vi "UHR-Fleezers Control (host) - 11.1.vi"() -> ()   [LabVIEW 2012] (continued)
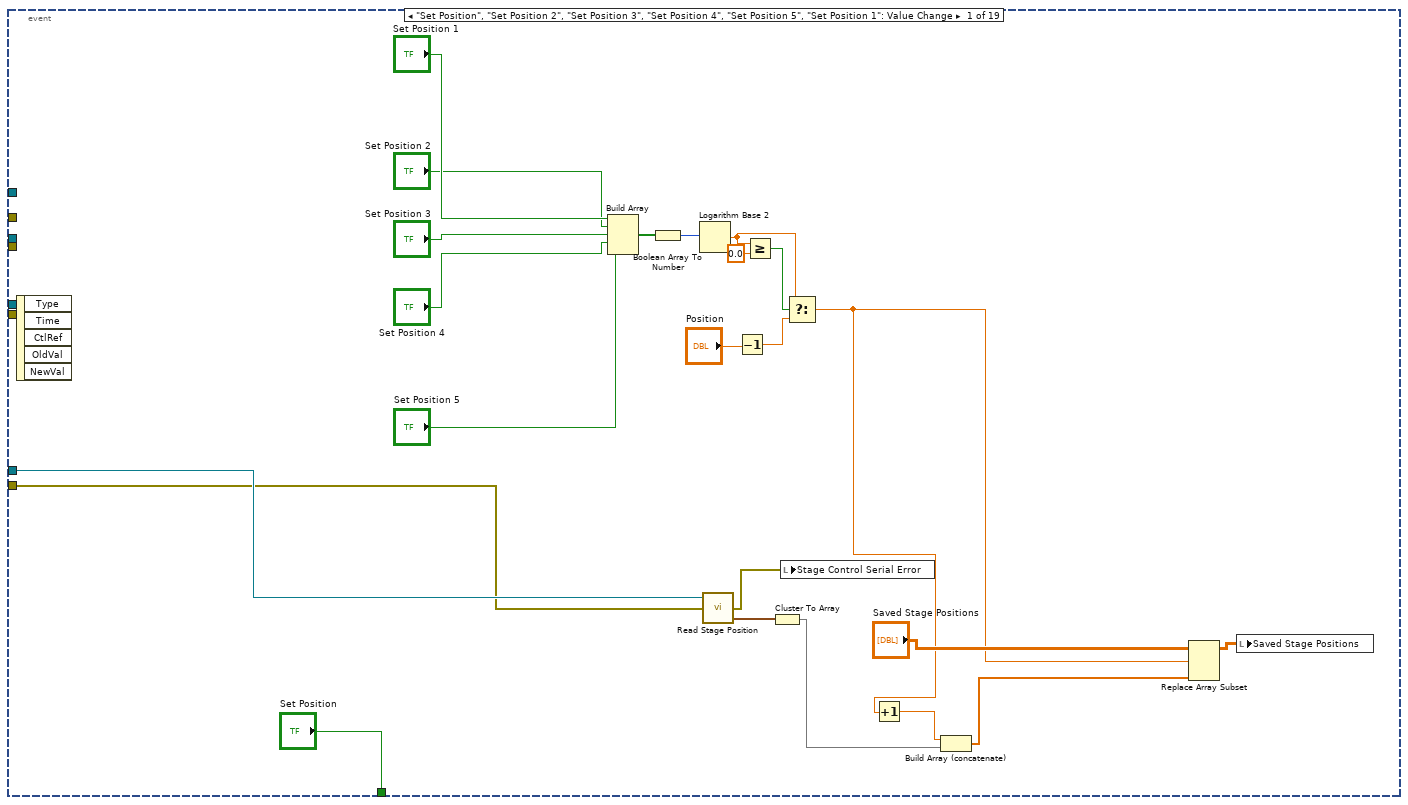
[diagram p2: hidden frame]
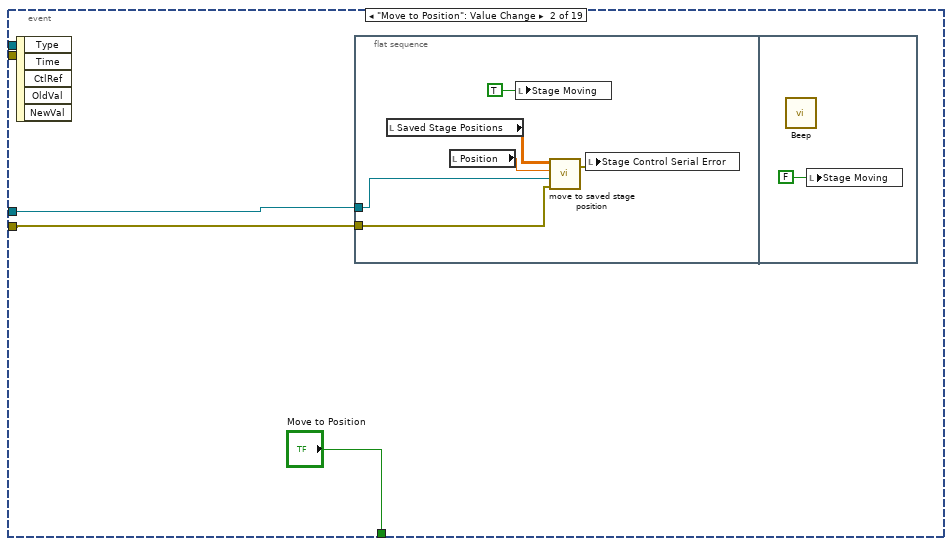
[diagram p3: hidden frame]
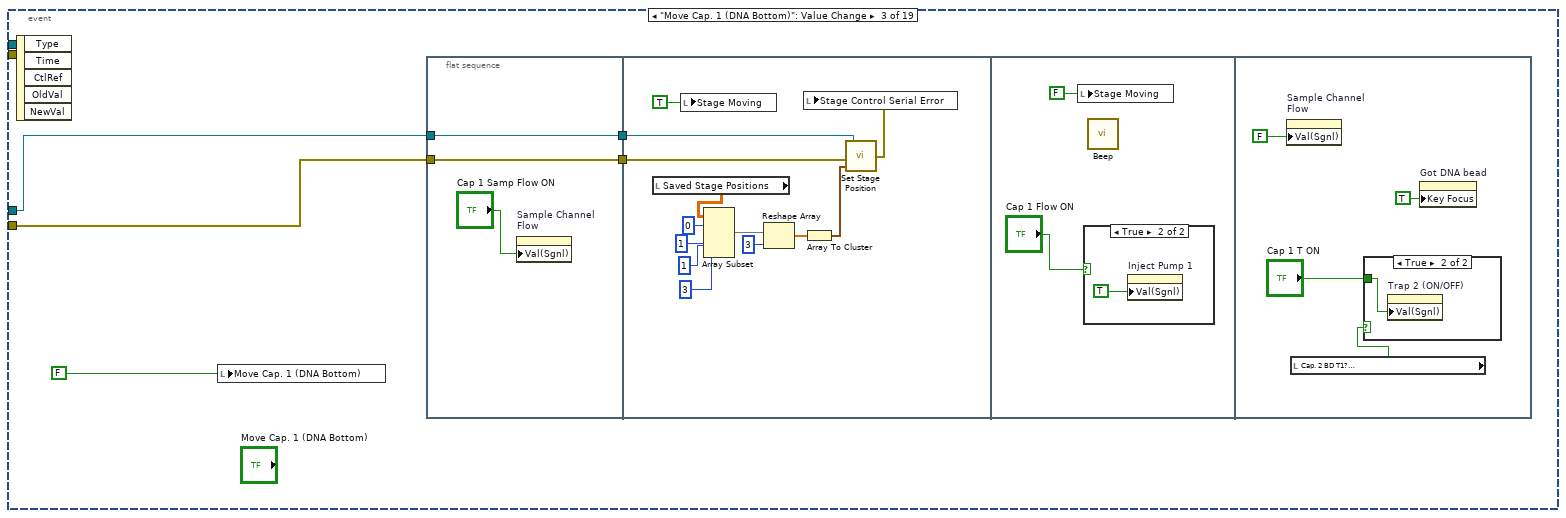
[diagram p4: hidden frame]
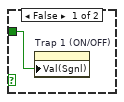
[diagram p6: hidden frame]
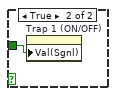
[diagram p8: hidden frame]
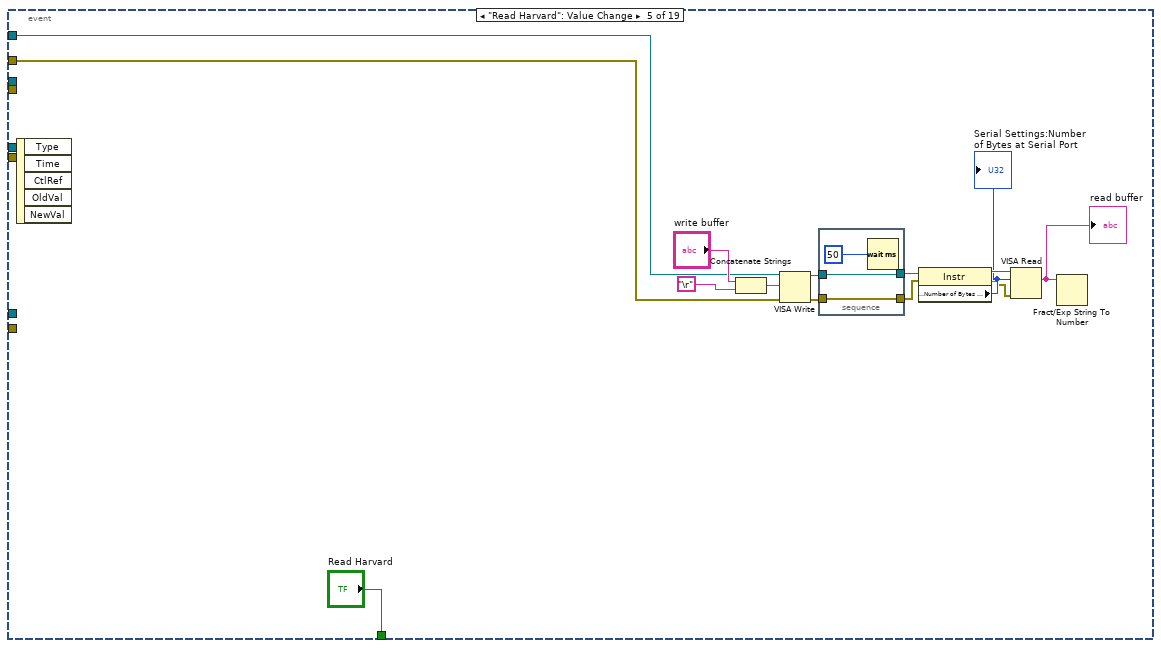
[diagram p9: hidden frame]
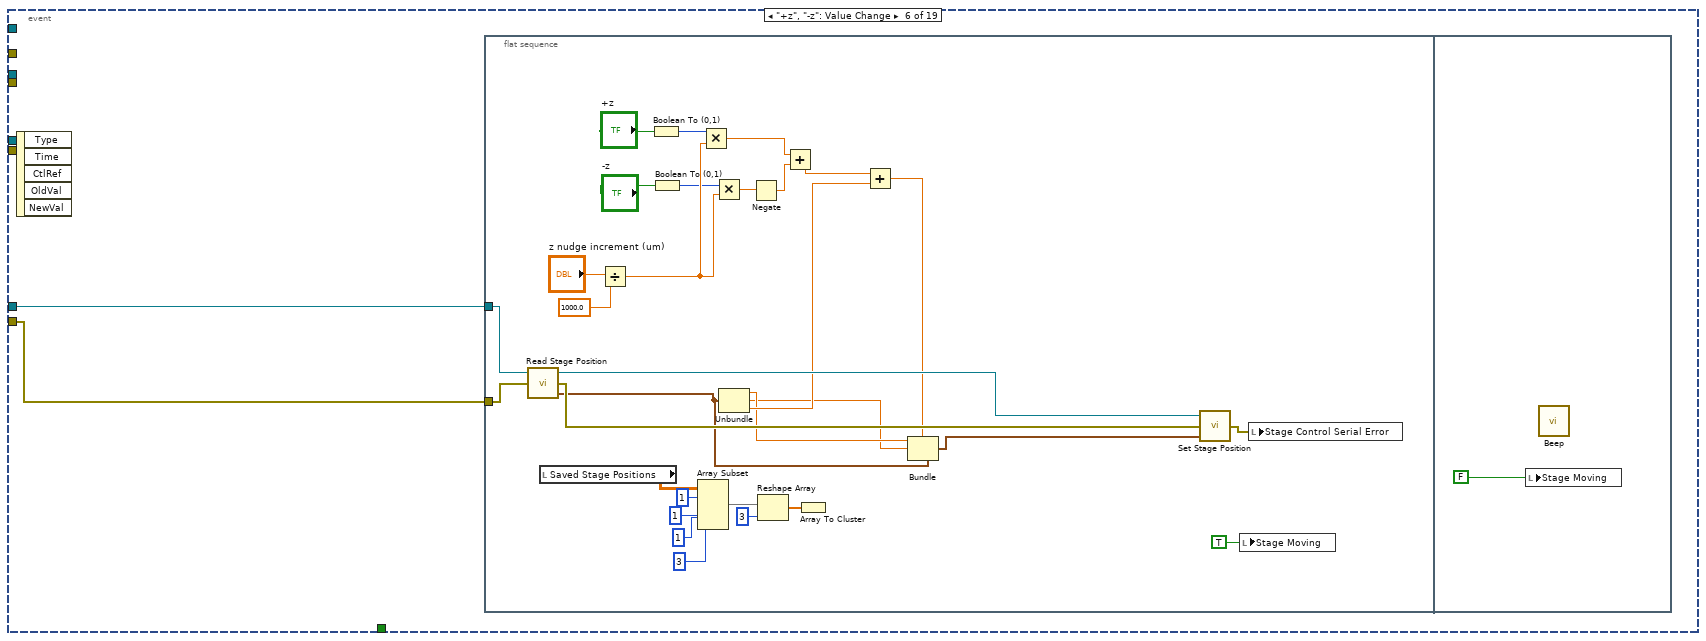
[diagram p10: hidden frame]
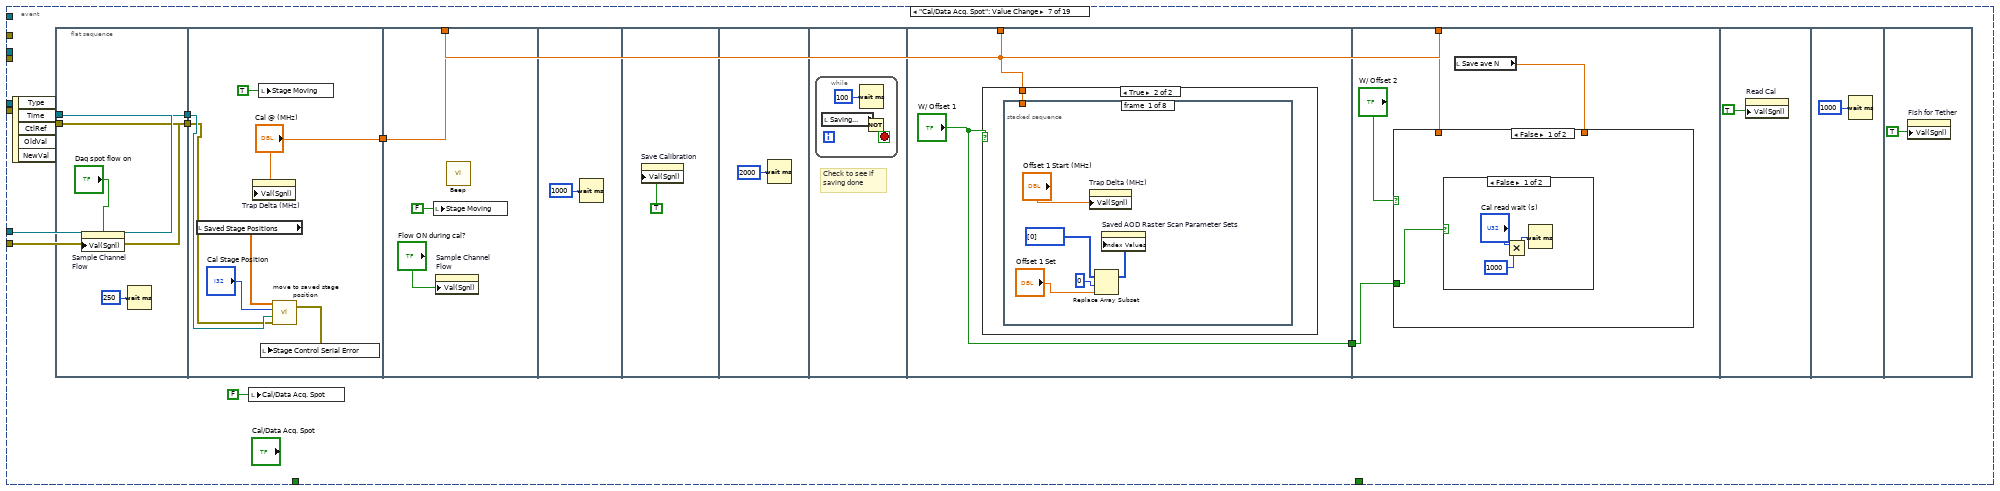
[diagram p11: hidden frame]
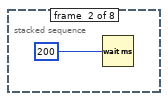
[diagram p13: hidden frame]
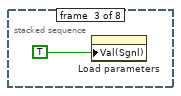
[diagram p14: hidden frame]
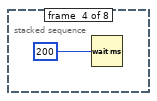
[diagram p15: hidden frame]
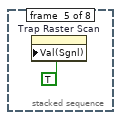
[diagram p16: hidden frame]
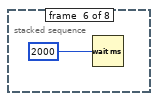
[diagram p17: hidden frame]
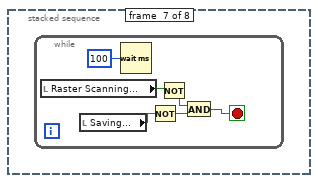
[diagram p18: hidden frame]
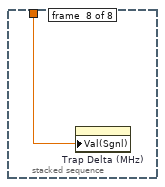
[diagram p19: hidden frame]
                                frame True {
                                n2888 = local read "Confocal Y 1 (V)"() -> (w4656:dbl)
                                n2889 = local read "Confocal X 1 (V)"() -> (w4655:dbl)
                                n2890 = property on="AO2" class="Slide (strict)"("Val(Sgnl)"=w4655) -> ()  [unwired: 2 in, 2 out]
                                n2891 = property on="AO1" class="Slide (strict)"("Val(Sgnl)"=w4656) -> ()  [unwired: 2 in, 2 out]
                                }
                                }
                                }
                                }
                                }
                                }
                                }
                                }
                                }
                                }
                                n2892 = local read "Time (s)"() -> (w4593:dbl)
                                n2893 = Subtract(x=w4594, y=w4593) -> (x-y=w4605:dbl)
                                n2894 = Number To Decimal String(number=w4605, width (-)=i16 0) -> (decimal integer string=w4603:string)
                                n2895 = Concatenate Strings(w4603, " s fluorescence event") -> (w4600:string)
                                n2896 = local read "Messages"() -> (w4601:string)
                                n2897 = local write "Duration (s)"(w4605) -> ()
                                n2898 = call "Update messages.vi"("Message to add"=w4600, "Old message string"=w4601) -> ("New message string"=w4599:string)
                                n2899 = local write "Messages"(w4599) -> ()
                                n2900 = call <vilib>:"Beep.vi"() -> ()  [unwired: 12 in]
                                n2901 = local write "Reset Force"(FALSE ("Force Reset")) -> ()
                                n2902 = local write "Fl. High"(TRUE ("Fl. High")) -> ()
                                n2903 = local write "Waiting"(TRUE ("Waiting")) -> ()
                                }
                                }
                                n2904 = node-c288() -> ()  [unwired: 1 in, 1 out]
                                }
                                n2905 = node-c288(w4572) -> ()  [unwired: 1 out]
                                }
                              }
                            }
                          }
                          n2906 = local read "Trap Delta (MHz)"() -> (w4484:dbl)
                          n2907 = local read "Trap Pos FB SP"() -> (w4482:fxp<+/-,16,1>)
                        }
                      }
                    }
                    frame True {
                      n2908 = flat-sequence {
                        tunnel: w4669 -> [w4679]
                        tunnel: [w4679] -> w4673
                        tunnel: w4672 -> [w4678]
                        tunnel: [w4678] -> w4671
                        tunnel: [w4677] -> w4670
                        tunnel: w4668 -> [w4676]
                        tunnel: [w4675] -> w4667
                        tunnel: w4664 -> [w4674]
                        tunnel: [w4674] -> w4663
                        tunnel: w4673 -> [w4749]
                        tunnel: w4671 -> [w4748]
                        tunnel: w4670 -> [w4747]
                        tunnel: w4667 -> [w4746]
                        tunnel: w4663 -> [w4745]
                        tunnel: [w4746] -> w4666
                        frame #0 {
                          n2909 = call <vilib>:"Beep.vi"() -> ()  [unwired: 3 in, 9 out]
                          n2910 = local write "Waiting"(FALSE ("Waiting")) -> ()
                          n2911 = Increment(x=w4676) -> (x+1=w4675:u8)
                          n2912 = case shown="\"Yank\"" w4678 {
                            tunnel: w4675 -> [_ _ w4685]
                            frame "Image" {
                              n2913 = property on="Confocal Image" class="Bool (strict)"("Val(Sgnl)"=TRUE ("Value (Signaling)")) -> ()  [unwired: 2 in, 2 out]
                            }
                            frame "Alarm", Default {
                            }
                            frame "Yank" {
                              n2914 = flat-sequence {
                                tunnel: w4685 -> [w4688]
                                tunnel: [w4687] -> w4684
                                tunnel: ["N Array El"] -> w4683
                                tunnel: w4684 -> [w4702]
                                tunnel: w4683 -> [w4698]
                                frame #0 {
                                n2915 = Multiply(x="Yank Delay (s)", y=1000.0) -> (x*y=w4691:dbl)
                                n2916 = Quotient & Remainder(x=w4688, y="N Array El") -> (x-y*floor(x/y)=w4687:u8)  [unwired: 1 out]
                                n2917 = Wait (ms)(milliseconds to wait=w4691) -> ()  [unwired: 1 out]
                                }
                                frame #1 {
                                n2918 = Random Number (0-1)() -> (number: 0 to 1=w4699:dbl)
                                n2919 = Multiply(x=w4698, y=w4699) -> (x*y=w4697:dbl)
                                n2920 = Round Toward -Infinity(1:w4697) -> (0:w4696:dbl)
                                n2921 = Select(t=w4696, s="Random Choice", f=w4702) -> (s? t:f=w4700:dbl)
                                n2922 = Select(t="Yank to Trap Delta (MHz)", s="Yank to which?", f="Yank to SP") -> (s? t:f=w4693:dbl[])
                                n2923 = Index Array(array=w4693, index=w4700) -> (element=w4703:dbl)
                                n2924 = case shown="False" "Yank to which?" {
                                tunnel: w4703 -> [w4704 w4730]
                                frame False {
                                n2925 = flat-sequence {
                                tunnel: w4704 -> [w4705]
                                frame #0 {
                                n2926 = property on="Trap Pos FB SP" class="DigNum (strict)"("Val(Sgnl)"=w4705) -> ()  [unwired: 2 in, 2 out]
                                }
                                frame #1 {
                                n2927 = Wait (ms)(milliseconds to wait=u32 700) -> ()  [unwired: 1 out]
                                }
                                frame #2 {
                                n2928 = local read "Action (%)"() -> (w4710:dbl)
                                n2929 = Absolute Value(x=w4710) -> (abs(x)=w4709:dbl)
                                n2930 = Greater?(x=w4709, y=70.0) -> (0:w4707:bool)
                                n2931 = property on="Remove Action Offset" class="Bool (strict)"("Val(Sgnl)"=w4707) -> ()  [unwired: 2 in, 2 out]
                                }
                                frame #3 {
                                n2932 = for {
                                N: 4 -> [_]
                                n2933 = flat-sequence {
                                frame #0 {
                                n2934 = Wait (ms)(milliseconds to wait=u32 500) -> ()  [unwired: 1 out]
                                }
                                frame #1 {
                                n2935 = local read "Action (%)"() -> (w4716:dbl)
                                n2936 = Absolute Value(x=w4716) -> (abs(x)=w4715:dbl)
                                n2937 = Greater?(x=w4715, y=70.0) -> (0:w4713:bool)
                                n2938 = property on="Remove Action Offset" class="Bool (strict)"("Val(Sgnl)"=w4713) -> ()  [unwired: 2 in, 2 out]
                                }
                                }
                                }
                                }
                                frame #4 {
                                n2939 = local read "Shift confocal"() -> (w4720:bool)
                                n2940 = local read "Mean"() -> (w4723:dbl)
                                n2941 = Greater?(x=w4723, y=11.0) -> (0:w4719:bool)
                                n2942 = Not(x=w4719) -> (.not. x?=w4718:bool)
                                n2943 = And(x=w4718, y=w4720) -> (x .and. y?=w4717:bool)
                                n2944 = And(x=w4719, y=w4720) -> (x .and. y?=w4721:bool)
                                n2945 = case shown="True" w4721 {
                                frame False {
                                }
                                frame True {
                                n2946 = local read "Confocal X 2 (V)"() -> (w4726:dbl)
                                n2947 = local read "Confocal Y 2 (V)"() -> (w4727:dbl)
                                n2948 = property on="AO2" class="Slide (strict)"("Val(Sgnl)"=w4726) -> ()  [unwired: 2 in, 2 out]
                                n2949 = property on="AO1" class="Slide (strict)"("Val(Sgnl)"=w4727) -> ()  [unwired: 2 in, 2 out]
                                }
                                }
                                n2950 = case shown="True" w4717 {
                                frame False {
                                }
                                frame True {
                                n2951 = local read "Confocal X 1 (V)"() -> (w4724:dbl)
                                n2952 = local read "Confocal Y 1 (V)"() -> (w4725:dbl)
                                n2953 = property on="AO1" class="Slide (strict)"("Val(Sgnl)"=w4725) -> ()  [unwired: 2 in, 2 out]
                                n2954 = property on="AO2" class="Slide (strict)"("Val(Sgnl)"=w4724) -> ()  [unwired: 2 in, 2 out]
                                }
                                }
                                }
                                frame #5 {
                                n2955 = Wait (ms)(milliseconds to wait=u32 1500) -> ()  [unwired: 1 out]
                                }
                                frame #6 {
                                n2956 = property on="Rem fb disp offset" class="Bool (strict)"("Val(Sgnl)"=TRUE ("Value (Signaling)")) -> ()  [unwired: 2 in, 2 out]
                                }
                                }
                                }
                                frame True {
                                n2957 = flat-sequence {
                                tunnel: w4730 -> [w4731]
                                frame #0 {
                                n2958 = property on="Trap Delta (MHz)" class="DigNum (strict)"("Val(Sgnl)"=w4731) -> ()  [unwired: 2 in, 2 out]
                                }
                                frame #1 {
                                n2959 = Wait (ms)(milliseconds to wait=u32 500) -> ()  [unwired: 1 out]
                                }
                                frame #2 {
                                n2960 = local read "Shift confocal"() -> (w4735:bool)
                                n2961 = local read "Mean"() -> (w4733:dbl)
                                n2962 = Greater?(x=w4733, y=11.0) -> (0:w4736:bool)
                                n2963 = Not(x=w4736) -> (.not. x?=w4737:bool)
                                n2964 = And(x=w4737, y=w4735) -> (x .and. y?=w4739:bool)
                                n2965 = And(x=w4736, y=w4735) -> (x .and. y?=w4738:bool)
                                n2966 = case shown="True" w4738 {
                                frame False {
                                }
                                frame True {
                                n2967 = local read "Confocal Y 2 (V)"() -> (w4743:dbl)
                                n2968 = local read "Confocal X 2 (V)"() -> (w4742:dbl)
                                n2969 = property on="AO1" class="Slide (strict)"("Val(Sgnl)"=w4743) -> ()  [unwired: 2 in, 2 out]
                                n2970 = property on="AO2" class="Slide (strict)"("Val(Sgnl)"=w4742) -> ()  [unwired: 2 in, 2 out]
                                }
                                }
                                n2971 = case shown="True" w4739 {
                                frame False {
                                }
                                frame True {
                                n2972 = local read "Confocal X 1 (V)"() -> (w4740:dbl)
                                n2973 = local read "Confocal Y 1 (V)"() -> (w4741:dbl)
                                n2974 = property on="AO2" class="Slide (strict)"("Val(Sgnl)"=w4740) -> ()  [unwired: 2 in, 2 out]
                                n2975 = property on="AO1" class="Slide (strict)"("Val(Sgnl)"=w4741) -> ()  [unwired: 2 in, 2 out]
                                }
                                }
                                }
                                }
                                }
                                }
                                }
                              }
                            }
                          }
                          n2976 = local read "Time (s)"() -> (w4677:dbl)
                          "Fl. High" <- TRUE ("Yanking")
                        }
                        frame #1 {
                          n2977 = local read "Auto F Reset"() -> (w4744:bool)
                          n2978 = case shown="True" w4744 {
                            tunnel: w4749 -> [_ w4753]
                            tunnel: w4748 -> [_ w4752]
                            tunnel: w4747 -> [_ w4751]
                            tunnel: w4745 -> [_ w4750]
                            frame False {
                            }
                            frame True {
                              n2979 = node-c288() -> (w4755:T21)  [unwired: 4 out]
                              n2980 = timed-loop {
                                timing: w4755 -> [_]
                                timing-out: [_] -> w4754
                                tunnel: w4753 -> [w4773]
                                tunnel: w4752 -> [w4772]
                                tunnel: w4751 -> [w4771]
                                tunnel: w4750 -> [w4770]
                                stop <- w4756 stop-if-true
                                n2981 = node-c288() -> ()  [unwired: 2 out]
                                n2982 = local read "Fl. Delta Thresh. (kHz)"() -> (w4764:dbl)
                                n2983 = local read "Fl. Triggered..."() -> (w4769:bool)
                                n2984 = local read "Delta Fl. 1"() -> (w4760:dbl)
                                n2985 = local read "Delta Fl. 2"() -> (w4758:dbl)
                                n2986 = local read "Stop All"() -> (w4767:bool)
                                n2987 = local read "APD to Watch"() -> (w4759:bool)
                                n2988 = Select(t=w4760, s=w4759, f=w4758) -> (s? t:f=w4757:dbl)
                                n2989 = Not(x=w4769) -> (.not. x?=w4768:bool)
                                n2990 = Multiply(x=w4764, y=1000.0) -> (x*y=w4763:dbl)
                                n2991 = Negate(x=w4763) -> (-x=w4762:dbl)
                                n2992 = Less?(x=w4757, y=w4762) -> (x < y?=w4766:bool)
                                n2993 = Compound Arithmetic op=OR(w4766, w4767, w4768, "Reset Force") -> (w4756:bool)
                                n2994 = case shown="True" w4756 {
                                tunnel: w4773 -> [_ w4788]
                                tunnel: w4772 -> [_ w4787]
                                tunnel: w4771 -> [_ w4777]
                                tunnel: w4770 -> [_ w4779]
                                frame False {
                                }
                                frame True {
                                n2995 = local read "Time (s)"() -> (w4778:dbl)
                                n2996 = case shown="\"Yank\"" w4787 {
                                tunnel: w4788 -> [_ w4791]
                                tunnel: w4779 -> [_ w4789]
                                frame "Image", Default {
                                }
                                frame "Yank" {
                                n2997 = flat-sequence {
                                tunnel: [w4797] -> w4792
                                tunnel: w4791 -> [w4797]
                                tunnel: [w4793] -> w4790
                                tunnel: w4789 -> [w4793]
                                tunnel: w4792 -> [w4800]
                                tunnel: w4790 -> [w4798]
                                frame #0 {
                                n2998 = local read "Yank Delay (s)"() -> (w4796:dbl)
                                n2999 = Multiply(x=w4796, y=1000.0) -> (x*y=w4794:dbl)
                                n3000 = Wait (ms)(milliseconds to wait=w4794) -> ()  [unwired: 1 out]
                                }
                                frame #1 {
                                n3001 = local read "Yank to which?"() -> (w4799:bool)
                                n3002 = case shown="False" w4799 {
                                tunnel: w4800 -> [_ w4827]
                                tunnel: w4798 -> [w4801 _]
                                frame False {
                                n3003 = flat-sequence {
                                tunnel: w4801 -> [w4802]
                                frame #0 {
                                n3004 = property on="Trap Pos FB SP" class="DigNum (strict)"("Val(Sgnl)"=w4802) -> ()  [unwired: 2 in, 2 out]
                                }
                                frame #1 {
                                n3005 = Wait (ms)(milliseconds to wait=u32 700) -> ()  [unwired: 1 out]
                                }
                                frame #2 {
                                n3006 = local read "Action (%)"() -> (w4807:dbl)
                                n3007 = Absolute Value(x=w4807) -> (abs(x)=w4806:dbl)
                                n3008 = Greater?(x=w4806, y=70.0) -> (0:w4804:bool)
                                n3009 = property on="Remove Action Offset" class="Bool (strict)"("Val(Sgnl)"=w4804) -> ()  [unwired: 2 in, 2 out]
                                }
                                frame #3 {
                                n3010 = for {
                                N: 4 -> [_]
                                n3011 = flat-sequence {
                                frame #0 {
                                n3012 = Wait (ms)(milliseconds to wait=u32 500) -> ()  [unwired: 1 out]
                                }
                                frame #1 {
                                n3013 = local read "Action (%)"() -> (w4813:dbl)
                                n3014 = Absolute Value(x=w4813) -> (abs(x)=w4812:dbl)
                                n3015 = Greater?(x=w4812, y=70.0) -> (0:w4810:bool)
                                n3016 = property on="Remove Action Offset" class="Bool (strict)"("Val(Sgnl)"=w4810) -> ()  [unwired: 2 in, 2 out]
                                }
                                }
                                }
                                }
                                frame #4 {
                                n3017 = local read "Shift confocal"() -> (w4818:bool)
                                n3018 = local read "Mean"() -> (w4820:dbl)
                                n3019 = Greater?(x=w4820, y=11.0) -> (0:w4817:bool)
                                n3020 = Not(x=w4817) -> (.not. x?=w4816:bool)
                                n3021 = And(x=w4817, y=w4818) -> (x .and. y?=w4815:bool)
                                n3022 = And(x=w4816, y=w4818) -> (x .and. y?=w4814:bool)
                                n3023 = case shown="True" w4815 {
                                frame False {
                                }
                                frame True {
                                n3024 = local read "Confocal Y 2 (V)"() -> (w4824:dbl)
                                n3025 = local read "Confocal X 2 (V)"() -> (w4823:dbl)
                                n3026 = property on="AO2" class="Slide (strict)"("Val(Sgnl)"=w4823) -> ()  [unwired: 2 in, 2 out]
                                n3027 = property on="AO1" class="Slide (strict)"("Val(Sgnl)"=w4824) -> ()  [unwired: 2 in, 2 out]
                                }
                                }
                                n3028 = case shown="True" w4814 {
                                frame False {
                                }
                                frame True {
                                n3029 = local read "Confocal X 1 (V)"() -> (w4821:dbl)
                                n3030 = local read "Confocal Y 1 (V)"() -> (w4822:dbl)
                                n3031 = property on="AO1" class="Slide (strict)"("Val(Sgnl)"=w4822) -> ()  [unwired: 2 in, 2 out]
                                n3032 = property on="AO2" class="Slide (strict)"("Val(Sgnl)"=w4821) -> ()  [unwired: 2 in, 2 out]
                                }
                                }
                                }
                                frame #5 {
                                n3033 = Wait (ms)(milliseconds to wait=u32 1500) -> ()  [unwired: 1 out]
                                }
                                frame #6 {
                                n3034 = property on="Rem fb disp offset" class="Bool (strict)"("Val(Sgnl)"=TRUE ("Value (Signaling)")) -> ()  [unwired: 2 in, 2 out]
                                }
                                }
                                }
                                frame True {
                                n3035 = flat-sequence {
                                tunnel: w4827 -> [w4828]
                                frame #0 {
                                n3036 = property on="Trap Delta (MHz)" class="DigNum (strict)"("Val(Sgnl)"=w4828) -> ()  [unwired: 2 in, 2 out]
                                }
                                frame #1 {
                                n3037 = Wait (ms)(milliseconds to wait=u32 500) -> ()  [unwired: 1 out]
                                }
                                frame #2 {
                                n3038 = local read "Shift confocal"() -> (w4834:bool)
                                n3039 = local read "Mean"() -> (w4836:dbl)
                                n3040 = Greater?(x=w4836, y=11.0) -> (0:w4833:bool)
                                n3041 = Not(x=w4833) -> (.not. x?=w4832:bool)
                                n3042 = And(x=w4833, y=w4834) -> (x .and. y?=w4831:bool)
                                n3043 = And(x=w4832, y=w4834) -> (x .and. y?=w4830:bool)
                                n3044 = case shown="True" w4831 {
                                frame False {
                                }
                                frame True {
                                n3045 = local read "Confocal Y 2 (V)"() -> (w4840:dbl)
                                n3046 = local read "Confocal X 2 (V)"() -> (w4839:dbl)
                                n3047 = property on="AO2" class="Slide (strict)"("Val(Sgnl)"=w4839) -> ()  [unwired: 2 in, 2 out]
                                n3048 = property on="AO1" class="Slide (strict)"("Val(Sgnl)"=w4840) -> ()  [unwired: 2 in, 2 out]
                                }
                                }
                                n3049 = case shown="True" w4830 {
                                frame False {
                                }
                                frame True {
                                n3050 = local read "Confocal Y 1 (V)"() -> (w4838:dbl)
                                n3051 = local read "Confocal X 1 (V)"() -> (w4837:dbl)
                                n3052 = property on="AO2" class="Slide (strict)"("Val(Sgnl)"=w4837) -> ()  [unwired: 2 in, 2 out]
                                n3053 = property on="AO1" class="Slide (strict)"("Val(Sgnl)"=w4838) -> ()  [unwired: 2 in, 2 out]
                                }
                                }
                                }
                                }
                                }
                                }
                                }
                                }
                                }
                                }
                                n3054 = local read "Messages"() -> (w4786:string)
                                n3055 = Subtract(x=w4778, y=w4777) -> (x-y=w4784:dbl)
                                "Duration (s)" <- w4784
                                n3056 = Number To Decimal String(number=w4784, width (-)=i16 0) -> (decimal integer string=w4782:string)
                                n3057 = Concatenate Strings(w4782, " s fluorescence event." ("string")) -> (w4780:string)
                                n3058 = call "Update messages.vi"("Message to add"=w4780, "Old message string"=w4786) -> ("New message string"=w4785:string)
                                n3059 = local write "Reset Force"(FALSE ("Reset Force")) -> ()
                                n3060 = local write "Waiting"(TRUE ("Waiting")) -> ()
                                n3061 = local write "Messages"(w4785) -> ()
                                n3062 = local write "Fl. High"(FALSE ("Fl. High")) -> ()
                                n3063 = call <vilib>:"Beep.vi"() -> ()  [unwired: 3 in, 9 out]
                                }
                                }
                                n3064 = node-c288() -> ()  [unwired: 2 out]
                              }
                              n3065 = node-c288(w4754) -> ()  [unwired: 1 out]
                            }
                          }
                        }
                      }
                      n3066 = local read "Trap Delta (MHz)"() -> (w4669:dbl)
                      n3067 = local read "Trap Pos FB SP"() -> (w4664:fxp<+/-,16,1>)
                    }
                  }
                }
                frame #1 {
                  n3068 = local read "Stop All"() -> (w4850:bool)
                  n3069 = local read "Fl. Triggered..."() -> (w4848:bool)
                  n3070 = Not(x=w4848) -> (.not. x?=w4849:bool)
                  n3071 = Or(x=w4849, y=w4850) -> (x .or. y?=w4847:bool)
                }
              }
              n3072 = case shown="True" w4441 {
                frame False {
                }
                frame True {
                  n3073 = local read "Confocal Y 1 (V)"() -> (w4451:dbl)
                  n3074 = local read "Confocal X 1 (V)"() -> (w4450:dbl)
                  n3075 = property on="AO2" class="Slide (strict)"("Val(Sgnl)"=w4450) -> ()  [unwired: 2 in, 2 out]
                  n3076 = property on="AO1" class="Slide (strict)"("Val(Sgnl)"=w4451) -> ()  [unwired: 2 in, 2 out]
                }
              }
              n3077 = case shown="True" w4441 {
                frame False {
                }
                frame True {
                  w4449 = FALSE ("Fl. High")
                  n3078 = local write "Waiting"(w4449) -> ()
                  n3079 = local write "Fl. High"(w4449) -> ()
                }
              }
              n3080 = node-c288() -> ()  [unwired: 2 out]
            }
            n3081 = node-c288(w4439) -> ()  [unwired: 1 out]
          }
        }
      }
      event "Stop All": Value Change {
        n3082 = event-data() -> ()  [unwired: 7 out]
        n3083 = local read "Stop All"() -> (w4855:bool)
      }
    }
    n3084 = node-c288() -> ()  [unwired: 2 out]
  }
  n3085 = node-c288(w96) -> ()  [unwired: 1 out]
  n3086 = node-c288(w98) -> ()  [unwired: 1 out]
  n3087 = node-c288(w83) -> ()  [unwired: 1 out]
  n3088 = property on="Saved trap pos" class="WFGraph (strict)"("Visible"=FALSE) -> ()  [unwired: 2 in, 2 out]
  n3089 = property on="Trap Delta Graph" class="WFGraph (strict)"("Visible"=TRUE) -> ()  [unwired: 2 in, 2 out]
  n3090 = local write "Trap pos"(FALSE ("Trap pos")) -> ()
  n3091 = local write "Offset (nm)"(0.0 ("Offset (nm)")) -> ()
  n3092 = local write "Bead Mean (nm)"(0.0 ("Bead Mean (nm)")) -> ()
  n3093 = VISA Close(VISA resource name=w87, error in (no error)=w86) -> (error out=w135:errorcluster)
  n3094 = call <vilib>:"Simple Error Handler.vi"("error in (no error)"=w135) -> ()  [unwired: 1 in, 8 out]
  n3095 = node-c288(w179) -> ()  [unwired: 1 out]
  n3096 = node-c288(w94) -> ()  [unwired: 1 out]
  n3097 = flat-sequence {
    tunnel: w273 -> [w4859]
    tunnel: w275 -> [w4860]
    tunnel: [w4858] -> w254
    tunnel: [w4857] -> w253
    tunnel: w235 -> [_]
    tunnel: w187 -> [_]
    tunnel: w100 -> [_]
    tunnel: w254 -> [w4861]
    tunnel: w253 -> [w4862]
    frame #0 {
      w4856 = FALSE ("AI to FIFO")
      n3098 = xnode "Read/Write Control"("FPGA VI Reference In"=w4860, "error in"=w4859, "AI to FIFO"=w4856, "APD to FIFO"=w4856) -> ("FPGA VI Reference Out"=w4858:T19, "error out"=w4857:errorcluster)
    }
    frame #1 {
      n3099 = xnode "Close FPGA VI Reference"("FPGA VI Reference In"=w4861, "error in"=w4862) -> ("error out"=→"error out":errorcluster)
    }
  }
